vi "AVS_Activate.vi"(7 "a_pDeviceId":u8[](array[numeric])) -> (4 "Output Value":i32, 8 "a_pDeviceId":u8[](array[numeric]))   [LabVIEW 2020]
uses:
  AvaSpecX64-DLL_9.4/avaspecx64.dll
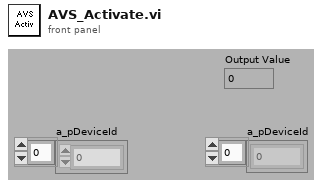
[diagram p1: front panel]
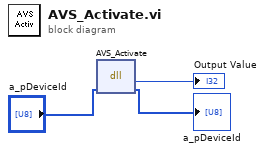
[diagram p0: block diagram]
diagram:
  n1 = dll-call lib="C:/AvaSpecX64-DLL_9.4/avaspecx64.dll" fn="AVS_Activate"("a_pDeviceId"="a_pDeviceId") -> ("return type"=→"Output Value":i32, "a_pDeviceId"=→"a_pDeviceId":u8[])  [unwired: 3 in, 2 out]
